vi "2 Global.vi"() -> ()   [LabVIEW 2011]
uses:
  2 Typedefs/UTM Location.ctl
  2 Typedefs/apparent wind.ctl
  2 Typedefs/Velocity.ctl
  2 Typedefs/heading.ctl
  2 Typedefs/generalized actuator status.ctl
  indicator LED.ctl
  2 Typedefs/generalized sensor status.ctl
panel:
  in  "Globals":T1(tab)
  in  "Which Boat Am I?":u16(ring) items=["Small RC", "Large RC", "Final Boat", "Simulator"]
  out "Direction Sensor Status":T2
  out "Location Sensor Status":T2
  out "Wind Sensor Status":T2
  out "Sail Actuator Status":T4
  out "Rudder Actuator Status":T4
  in  "Battery Voltage":dbl
  in  "Robot\nHeading":T5 format="%05.1f"
  in  "Robot UTM Location":T6
  in  "Robot Velocity":T7
  in  "Absolute Wind":cluster{"East":dbl, "North":dbl}
  in  "Apparent Wind\nDirection":dbl
  in  "Apparent Wind\nVelocity":dbl
  in  "Apparent Wind":T8
  in  "Rudder Angle":dbl
  in  "Sail Position":dbl
  # "All distances in meters\nAll angles in degrees, clockwise with 0 being positive North\nAll speeds in meters per second\nX-Y make a right handed coordinate system with Z pointing up\nPositive Rudder angle makes the boat turn right\nLocation Coordinates are in UTM format"
  # "As Measured"
  # "Path Planning"
  # "Mission Definition Stuff Goes HERE"
  # "To Boat"
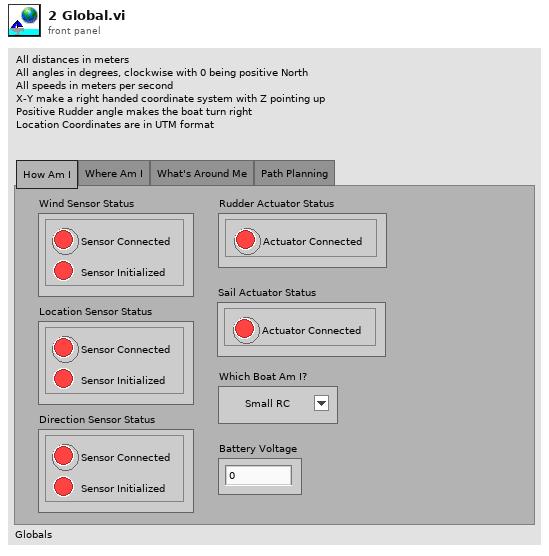
[diagram p1: front panel]
types:
  T1 = enum32{"How Am I", "Where Am I", "What's Around Me", "Path Planning"}
  T2 = typedef "generalized sensor status.ctl" = cluster{"Sensor Connected":T3, "Sensor Initialized":T3}
  T3 = typedef "indicator LED.ctl" = bool
  T4 = typedef "generalized actuator status.ctl" = cluster{"Actuator Connected":T3}
  T5 = typedef "heading.ctl" = dbl
  T6 = typedef "UTM Location.ctl" = cluster{"UTM Zone":dbl, "Hemisphere":enum16{"North", "South"}, "East":dbl, "North":dbl}
  T7 = typedef "Velocity.ctl" = cluster{"East":dbl, "North":dbl}
  T8 = typedef "apparent wind.ctl" = cluster{"Toward Fore":dbl, "Toward Starboard":dbl}
diagram:
